vi "sr830_convert_time_constant.vi"(3 "Time constant code":dbl) -> (1 "time constant  in ms":dbl)   [LabVIEW 2018]
panel:
  out "x = even?":bool
  # "Calculates the time constant in ms from the code obtained from SR830"
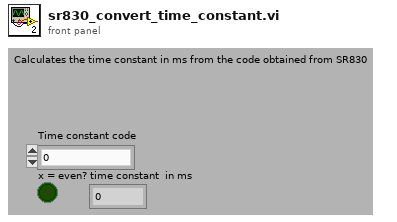
[diagram p1: front panel]
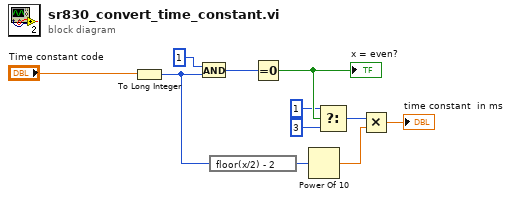
[diagram p0: block diagram]
diagram:
  n1 = To Long Integer(number="Time constant code") -> (32bit integer=w5:i32)
  n2 = And(x=1, y=w5) -> (x .and. y?=w10:i32)
  n3 = expression code="floor(x/2) - 2"(w5) -> (w3:i32)
  n4 = Equal To 0?(x=w10) -> (x = 0?=w9:bool)
  "x = even?" <- w9
  n5 = Power Of 10(x=w3) -> (10^x=w2:dbl)
  n6 = Select(t=1, s=w9, f=3) -> (s? t:f=w6:i32)
  n7 = Multiply(x=w6, y=w2) -> (x*y=→"time constant  in ms":dbl)
